vi "Version String to Build Spec Version.vi"(1 "Package Version":string) -> (0 "Build Specification Version":T1)   [LabVIEW 2019, in "PostBuildSupport.lvclass"]
uses:
  <vilib>/AppBuilder/AB_API_Simple/Build Specification Version.ctl
  PostBuildSupport.lvclass
  <vilib>/AppBuilder/AB_API_Simple/NI_App_Builder_API.lvlib
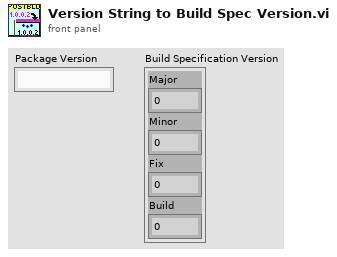
[diagram p1: front panel]
types:
  T1 = typedef "NI_App_Builder_API.lvlib/Build Specification Version.ctl" = cluster{"Major":u16, "Minor":u16, "Fix":u16, "Build":u16}
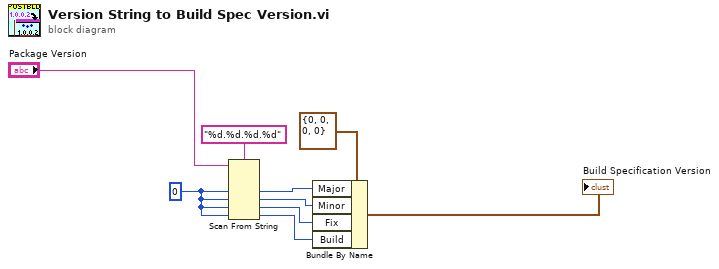
[diagram p0: block diagram]
diagram:
  w9 = u16 0 ("default value 1")
  n1 = Scan From String(format string="%d.%d.%d.%d", input string="Package Version", default 1=w9, default 2=w9, default 3=w9, default 4=w9) -> (output 1=w4:u16, output 2=w1:u16, output 3=w5:u16, output 4=w2:u16)  [unwired: 2 in, 3 out]
  n2 = Bundle By Name(cluster=T1 {"Major"=0, "Minor"=0, "Fix"=0, "Build"=0} ("Build Specification Version"), "Major"=w4, "Minor"=w1, "Fix"=w5, "Build"=w2) -> (→"Build Specification Version":T1)
